vi "GLdrv_FILE_RD.vi"(0 "Connection ID":T1, 5 "Folder":string, 11 "error in (no error)":errorcluster) -> (4 "Connection ID Out":T1, 15 "error out":errorcluster)   [LabVIEW 2017, in "GL860_Driver.lvlib"]
doc: "ディレクトリの削除を行います\n例) :FILE:RD “\\SD\\FOLDER3\\”"
uses:
  GL860_Driver.lvlib
  ConnectionID.ctl
  GLdrv_RW.ctl
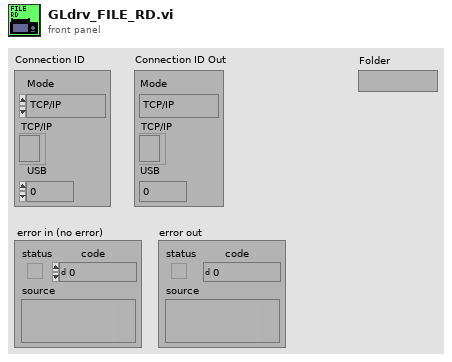
[diagram p1: front panel]
types:
  T1 = typedef "ConnectionID.ctl" = cluster{"Mode":enum16{"TCP/IP", "USB"}, "TCP/IP":refnum<k5>, "USB":i32}
  T2 = typedef "GLdrv_RW.ctl" = enum16{"Auto", "Read", "Write", "Buffer"}
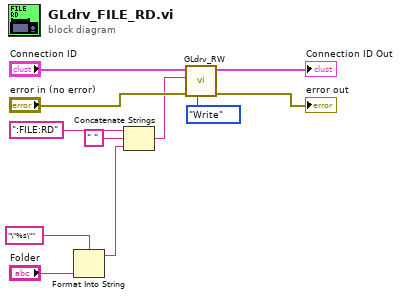
[diagram p0: block diagram]
diagram:
  n1 = Format Into String(format string="\"%s\"" ("Param"), "Folder") -> (resulting string=w1:string)  [unwired: 2 in, 1 out]
  n2 = Concatenate Strings(":FILE:RD" ("Command"), " " ("string"), w1) -> (w3:string)
  n3 = call "GLdrv_RW.vi"("Mode(read)"=GLdrv_RW."Write", "error in (no error)"="error in (no error)", "data in"=w3, "Connection ID"="Connection ID") -> ("error out"=→"error out":errorcluster, "Connection ID Out"=→"Connection ID Out":T1)  [unwired: 3 in, 3 out]
